vi "read.vi"(0 "连接ID":refnum<k5>) -> (1 "连接ID输出":refnum<k5>, 2 "数据输出":string)   [LabVIEW 2017]
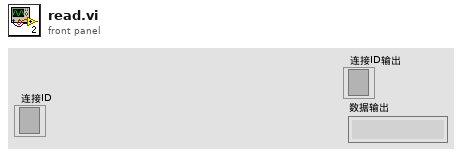
[diagram p1: front panel]
types:
  T1 = enum16{"Standard", "Buffered", "CRLF", "Immediate"}
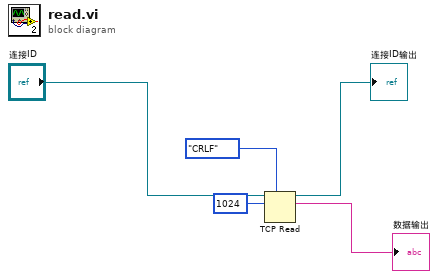
[diagram p0: block diagram]
diagram:
  n1 = TCP Read(connection ID="连接ID", bytes to read=1024 ("读取的字节"), 7:T1."CRLF" ("模式（标准）")) -> (connection ID out=→"连接ID输出":refnum<k5>, data out=→"数据输出":string)  [unwired: 2 in, 1 out]
